vi "Read (1D I16).vi"(7 "count (-1: all)":i64=-1 format="%d elements", 8 "error in (no error)":errorcluster, 9 "offset (0)":u64 format="%d bytes", 10 "buffer in":i16[](array[numeric]), 11 "Pointer in":refnum<class "Pointer.lvclass">) -> (0 "error out":errorcluster, 1 "offset out":u64 format="%d bytes", 2 "buffer out":i16[](array[numeric]), 3 "Pointer out":refnum<class "Pointer.lvclass">)   [LabVIEW 2016, in "Memory Manager.lvlib" / "Pointer.lvclass"]
doc: "Reads <b>count</b> elements from the address specified by <b>pointer + offset</b> into the provided <b>buffer</b>.\n\n<b>Note:</b> This VI is <b>safe</b>.\n\nSafe means that this function evaluates the size parameter of <b>pointer</b> to ensure that is inbounds of allocated memory before peforming a memory read/write. Reading/writing more data to a pointer than it has allocated can corrupt or crash LabVIEW."
uses:
  Pointer.lvclass
  Pointer.lvclass/Pointer.ctl
  Get Address.vi
  Errors.vi
  Null Pointer.vi
  Out of Bounds.vi
  Get Size.vi
  Count to Size.vi
  Create Error.vi
  Write Pointer Size.vi
  Get Error Info.vi
  VIs/Source.Write.String.vi
  VIs/Source.Write.Scalar.Base10.vi
  VIs/Source.Write.Scalar.Base10 (U64).vi
  VIs/Error Cluster.Set VI Source.vi
  VIs/Error Cluster.Set Code.vi
  VIs/Error Cluster.Set Status.vi
  VIs/New Error Cluster Constant.vi
  VIs/New Error Cluster Constant (512B).vi
  Constants/Constants.vi
  Constants/Library Name.vi
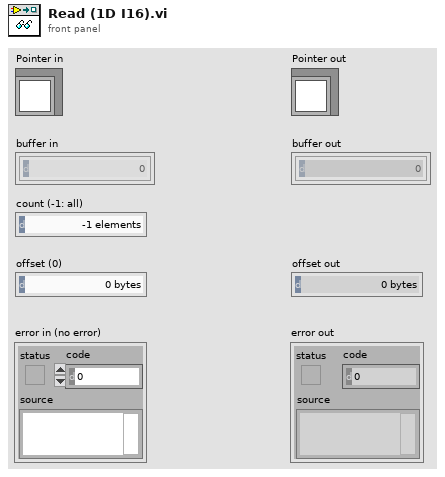
[diagram p1: front panel]
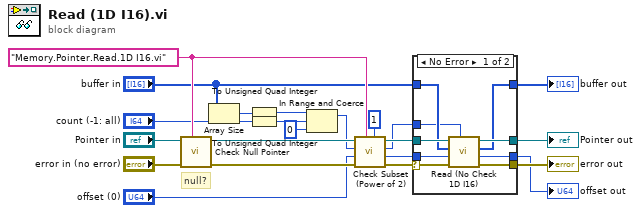
[diagram p0: block diagram]
diagram:
  w11 = "Memory.Pointer.Read.1D I16.vi" ("source vi name")
  # "null?"
  n1 = call "Check Null Pointer.vi"("source vi name"=w11, "error in (no error)"="error in (no error)", "Pointer in"="Pointer in") -> ("error out"=w14:errorcluster, "Pointer out"=w13:refnum<class "Pointer.lvclass">)  [unwired: 7 in]
  n2 = Array Size(array="buffer in") -> (size(s)=w10:i32)
  n3 = To Unsigned Quad Integer(1:w10) -> (0:w7:u64)
  n4 = To Unsigned Quad Integer(1:"count (-1: all)") -> (0:w8:u64)
  n5 = In Range and Coerce(upper limit=w7, x=w8, lower limit=u64 0) -> (coerced(x)=w5:u64)  [unwired: 1 out]
  n6 = call "Check Subset (Power of 2).vi"("power of 2"=i16 1, "source vi name"=w11, "error in (no error)"=w14, "offset (0)"="offset (0)", "count"=w5, "Pointer in"=w13) -> ("error out"=w22:errorcluster, "offset out"=w20:u64, "count"=w1:u64, "Pointer out"=w21:refnum<class "Pointer.lvclass">)  [unwired: 2 in]
  n7 = case shown="No Error" w22 {
    selector: w22 -> [w31 w34]
    tunnel: w21 -> [w29 w33]
    tunnel: w20 -> [w30 w35]
    tunnel: "buffer in" -> [w25 w32]
    tunnel: [w28 w34] -> w17
    tunnel: [w27 w33] -> w16
    tunnel: [w26 w35] -> w2
    tunnel: [w24 w32] -> w18
    tunnel: w1 -> [w23 _]
    frame No Error {
      n8 = call "Read (No Check 1D I16).vi"("count"=w23, "error in (no error)"=w31, "offset (0)"=w30, "buffer in"=w25, "Pointer in"=w29) -> ("error out"=w28:errorcluster, "offset out"=w26:u64, "buffer out"=w24:i16[], "Pointer out"=w27:refnum<class "Pointer.lvclass">)  [unwired: 3 in]
    }
    frame Error {
    }
  }
  "error out" <- w17
  "Pointer out" <- w16
  "buffer out" <- w18
  "offset out" <- w2
